vi "XferCoils.vi"(0 "Strings in":string[](array[string])=["C:\\CuspControl\\GPIB and Network\\Cusp\\Dummyfile.txt", "6723"], 1 "Dubs in":dbl[](array[numeric])=[0.0]) -> ()   [LabVIEW 2018]
uses:
  <vilib>/DAQmx/write.llb/DAQmx Write (Analog DBL 1Chan 1Samp).vi
  <vilib>/DAQmx/create/channels.llb/DAQmx Create Channel (AO-Voltage-Basic).vi
  <vilib>/DAQmx/miscellaneous.llb/DAQmx Fill In Error Info.vi
panel:
  in  "Default Voltages (2,3,5)":dbl[](array[numeric])=[2.0, 3.0, 5.0]
  in  "ON":bool
  in  "Min allowed":dbl[](array[numeric])=[0.0, 0.0, 0.0]
  in  "Max allowed":dbl[](array[numeric])=[10.0, 10.0, 5.0]
  in  "Applied voltages (2,3,5)":dbl[](array[numeric])=[0.0, 0.0, 0.0]
  out "Elapsed time (ms)":u32=5
  in  "subvi":bool=TRUE
  out "error out":errorcluster
  in  "AO2 name":string="6723"
  in  "ao lines":string[](array[string])=["/ao15", "/ao16", "/ao17"]
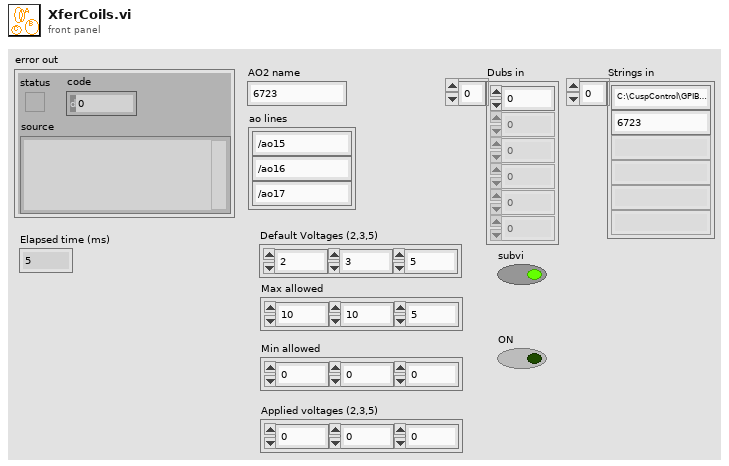
[diagram p1: front panel]
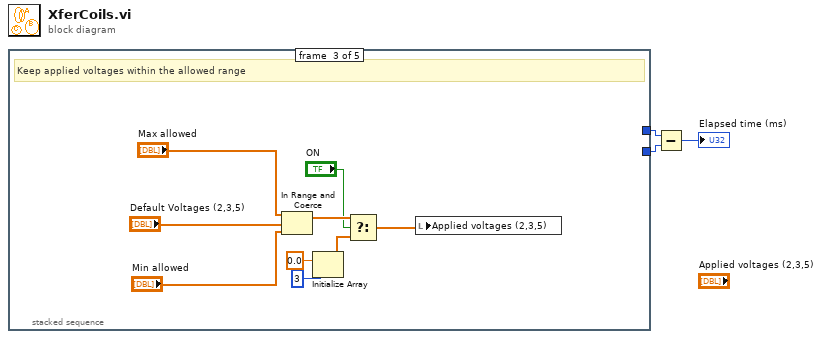
[diagram p0: block diagram]
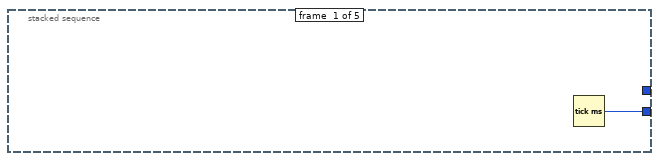
[diagram p2: hidden frame]
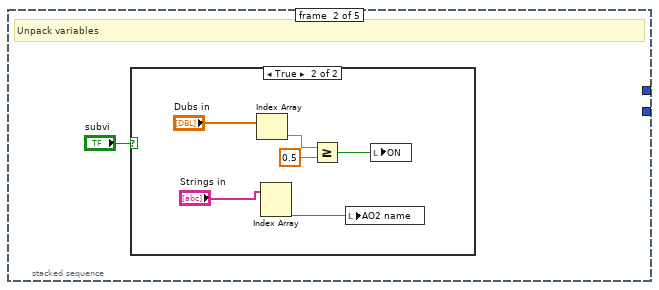
[diagram p3: hidden frame]
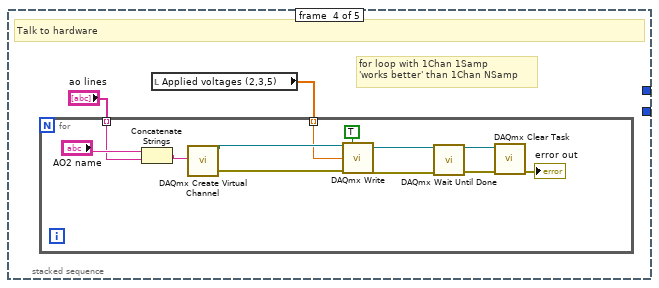
[diagram p5: hidden frame]
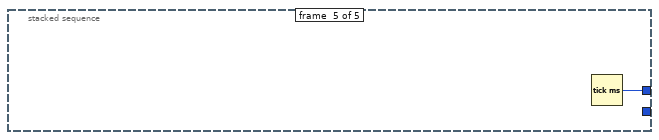
[diagram p6: hidden frame]
diagram:
  n1 = stacked-sequence {
    tunnel: [w4 _ _ _ _] -> w2
    tunnel: [_ _ _ _ w35] -> w3
    frame #0 {
      n2 = Tick Count (ms)() -> (millisecond timer value=w4:u32)
    }
    frame #1 {
      # "Unpack variables"
      n3 = case shown="True" "subvi" {
        frame False {
        }
        frame True {
          n4 = Index Array(array="Dubs in") -> (element=w8:dbl)  [unwired: 1 in]
          n5 = Index Array(array="Strings in") -> (element #2=w10:string)  [unwired: 2 in, 1 out]
          n6 = Greater Or Equal?(x=w8, y=0.5) -> (x >= y?=w6:bool)
          n7 = local write "AO2 name"(w10) -> ()
          n8 = local write "ON"(w6) -> ()
        }
      }
    }
    frame #2 {
      # "Keep applied voltages within the allowed range"
      n9 = In Range and Coerce(upper limit="Max allowed", x="Default Voltages (2,3,5)", lower limit="Min allowed") -> (coerced(x)=w18:dbl[])  [unwired: 1 out]
      n10 = Initialize Array(0.0 ("element"), 3 ("dimension size")) -> (w16:dbl[])
      n11 = Select(t=w18, s="ON", f=w16) -> (s? t:f=w17:dbl[])
      n12 = local write "Applied voltages (2,3,5)"(w17) -> ()
    }
    frame #3 {
      # "for loop with 1Chan 1Samp \n'works better' than 1Chan NSamp"
      # "Talk to hardware"
      n13 = local read "Applied voltages (2,3,5)"() -> (w22:dbl[])
      n14 = for {
        tunnel: w22 -> [w25] mode=indexing
        tunnel: "ao lines" -> [w23] mode=indexing
        n15 = Concatenate Strings("AO2 name", w23) -> (w30:string)
        n16 = call-poly <vilib>:"DAQmx Create Virtual Channel.vi"("physical channels"=w30) -> ("task out"=w27:refnum<k21>, "error out"=w26:errorcluster)  [unwired: 13 in]
        n17 = call-poly <vilib>:"DAQmx Write.vi"("task/channels in"=w27, "auto start"=TRUE, "data"=w25, "error in"=w26) -> ("task out"=w32:refnum<k21>, "error out"=w31:errorcluster)  [unwired: 9 in, 1 out]
        n18 = call <vilib>:"DAQmx Wait Until Done.vi"("task/channels in"=w32, "error in"=w31) -> ("task out"=w34:refnum<k21>, "error out"=w33:errorcluster)  [unwired: 12 in]
        n19 = call <vilib>:"DAQmx Clear Task.vi"("task in"=w34, "error in"=w33) -> ("error out"=→"error out":errorcluster)  [unwired: 13 in]
      }
    }
    frame #4 {
      n20 = Tick Count (ms)() -> (millisecond timer value=w35:u32)
    }
  }
  n21 = Subtract(x=w3, y=w2) -> (x-y=→"Elapsed time (ms)":u32)
